vi "SensorTest-05-2017.vi"() -> ()   [LabVIEW 2010]
uses:
  <vilib>/userDefined/High Color/nirio_resource_hc.ctl
  <vilib>/rvi/interface/nirviOpenFPGA/nirviOpenFPGA.xnode
  C:/Users/HAGAR-IV/Desktop/Zeugs/markus/version feb 2012/FPGA Bitfiles/pertrasgcfpga2_FPGATarget_FPGA-TrapTest-05_C2F74D86.lvbitx
  C:/Users/HAGAR-IV/Desktop/Zeugs/Johnny/pertrasgc fpga/FPGA-TrapTest-05-2017.vi
  <vilib>/rvi/ClientSDK/nirviWhatTheDeviceIsDoing.ctl
  <vilib>/rvi/interface/nirviReadWriteControl/nirviReadWriteControl.xnode
  <vilib>/rvi/interface/common/niFpgaNodeNameForErrorReporting.ctl
  <vilib>/rvi/errors/niLvFpgaWhatHappensToTopLevelVI.ctl
  <vilib>/rvi/interface/nirviMethod/nirviMethod.xnode
  <vilib>/rvi/interface/nirviCloseFPGA/nirviCloseFPGA.xnode
  <vilib>/FPGAPlugInAG/cRIO-9114/niLvFpga_Open_cRIO-9114.vi
  <vilib>/Utility/error.llb/Error Cluster From Error Code.vi
  <vilib>/rvi/errors/niLvFpgaAdjustHostInterfaceError.vi
  <vilib>/FPGAPlugInAG/cRIO-9114/niLvFpga_Close_cRIO-9114.vi
  NiFpgaLv.dll
panel:
  out "MainCol2b":dbl format="%.23g"
  out "MainCol2a":dbl format="%.23g"
  out "MainCol1b":dbl format="%.23g"
  out "MainCol1a":dbl format="%.23g"
  out "PreCol2":dbl format="%.23g"
  out "PreCol1":dbl format="%.23g"
  out "Thermoelement":dbl format="%.23g"
  out "PTStirling":dbl format="%.23g"
  out "MesswertTrap2":dbl format="%.23g"
  out "MesswertTrap1":dbl format="%.23g"
  out "MesswertTrap2":dbl[](graph)
  out "MesswertTrap1":dbl[](graph)
  in  "Löschen":bool
  in  "Messwerte":i32=10
  in  "5Van(us)":u16=5500
  in  "Periode(us)":u32=100000
  in  "Warten(us)":u16=5000
  in  "zwischenMesswerten(us)":u16=10
  in  "stop":bool
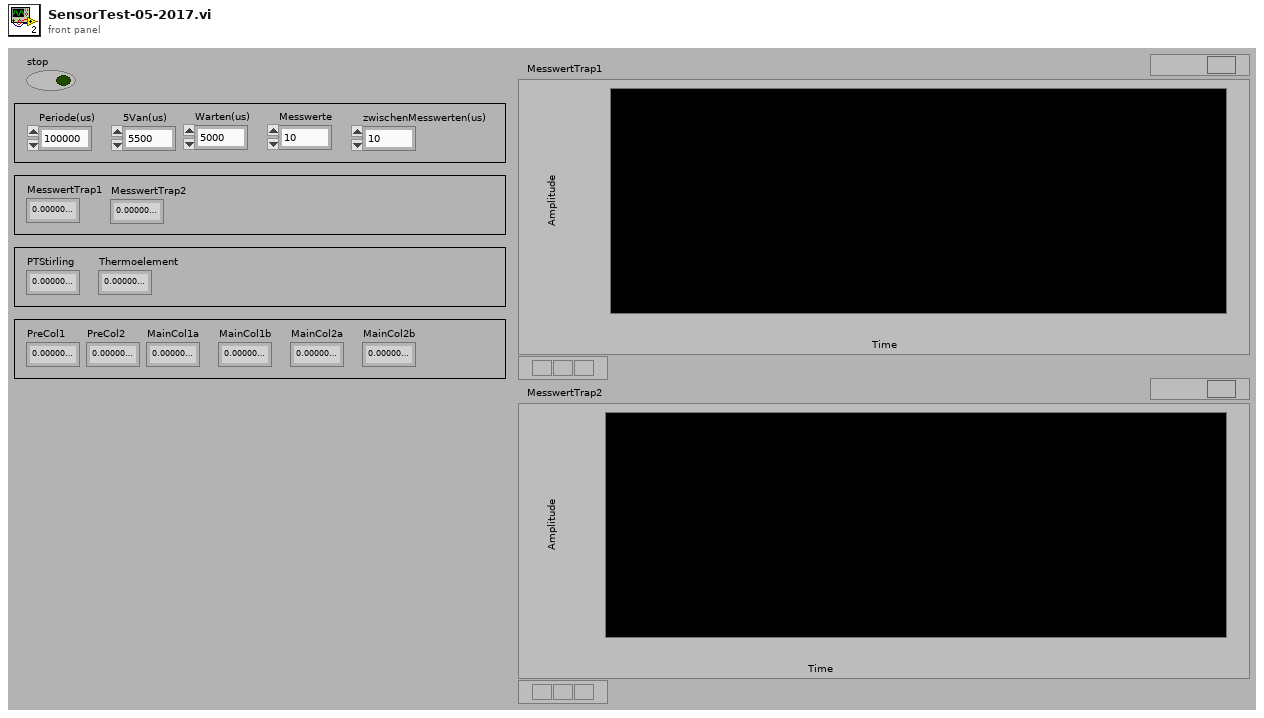
[diagram p1: front panel]
types:
  T1 = typedef "niFpgaNodeNameForErrorReporting.ctl" = enum16{"Open FPGA VI Reference", "Read/Write Control", "Invoke Method: Abort", "Invoke Method: Acknowledge IRQ", "Invoke Method: Download", "Invoke Method: FIFO.Configure", "Invoke Method: FIFO.Read", "Invoke Method: FIFO.Start", "Invoke Method: FIFO.Stop", "Invoke Method: FIFO.Write", "Invoke Method: Reset", "Invoke Method: Run", "Invoke Method: Wait on IRQ", "Close FPGA VI Reference"}
  T2 = typedef "niLvFpgaWhatHappensToTopLevelVI.ctl" = enum16{"top level VI scripted behind XNode", "top level VI inlined behind XNode"}
  T3 = cluster{"proportional gain (Kc)":fxp<+/-,16,8>, "integral gain (Kc*Ts/Ti)":fxp<+/-,16,8>, "derivative gain (Kc*Td/Ts)":fxp<+/-,16,8>}
  T4 = cluster{"[0]":dbl, "[1]":dbl, "[2]":dbl, "[3]":dbl, "[4]":dbl, "[5]":dbl, "[6]":dbl, "[7]":dbl, "[8]":dbl, "[9]":dbl}
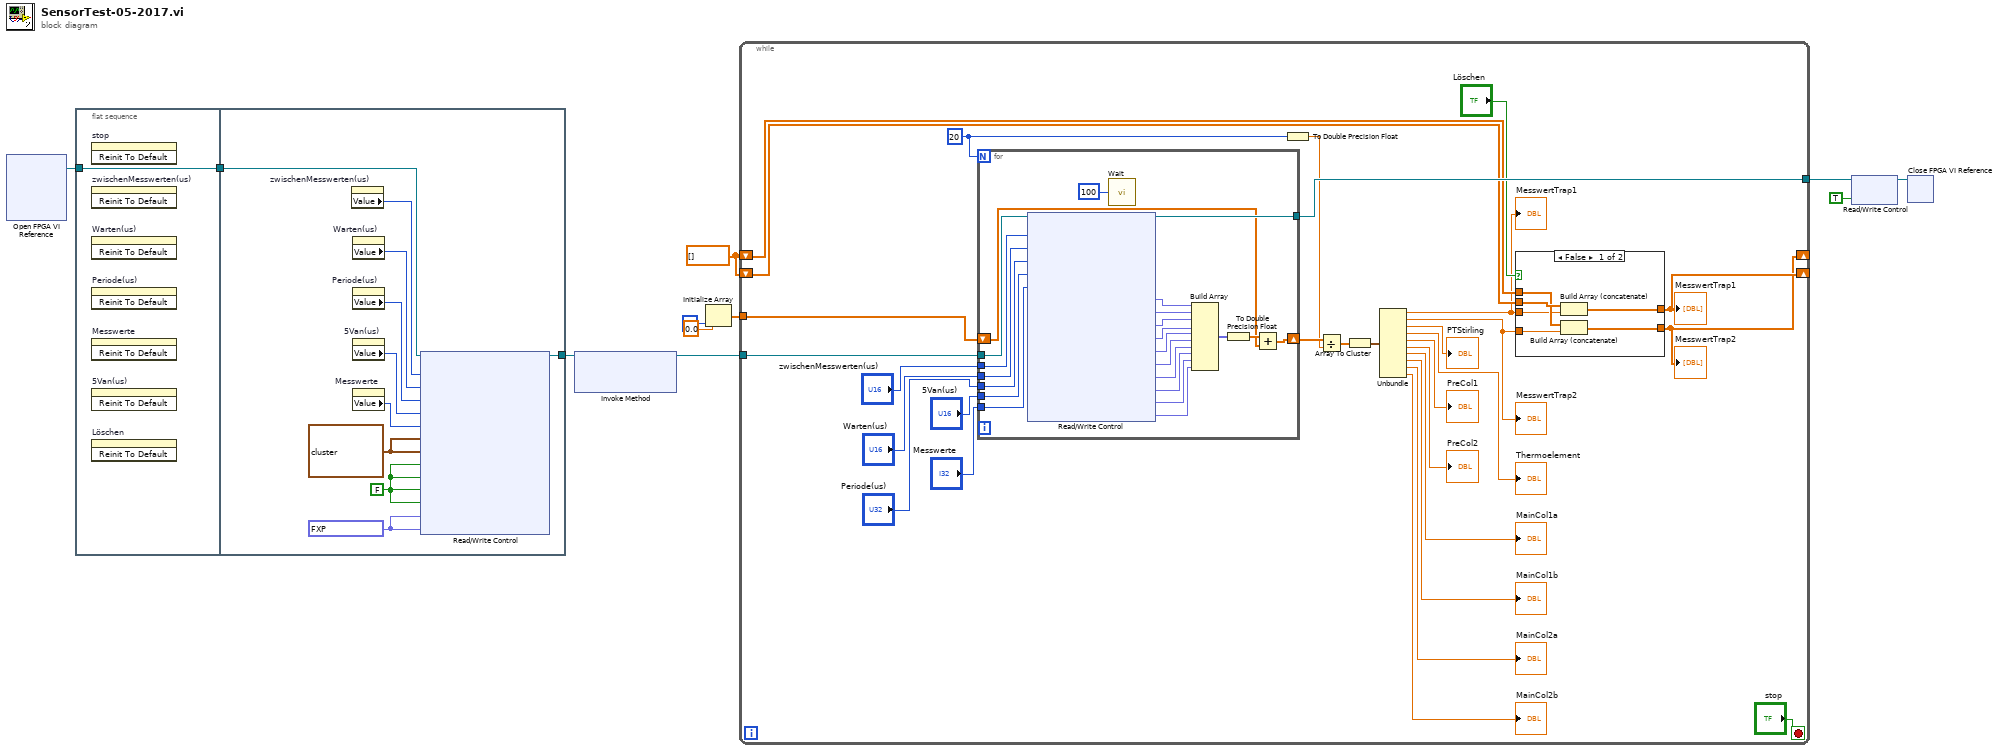
[diagram p0: block diagram]
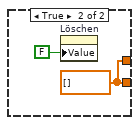
[diagram p2: hidden frame]
diagram:
  w4 = dbl[] []
  n1 = xnode "Open FPGA VI Reference"() -> ("FPGA VI Reference Out"=w11:refnum<k20>)  [unwired: 2 in, 1 out]
  n2 = flat-sequence {
    tunnel: w11 -> [w12]
    tunnel: [w12] -> w5
    tunnel: [w21] -> w10
    tunnel: w5 -> [w22]
    frame #0 {
      n3 = invoke on="stop" class="Bool (strict)" method="Reinit To Default"() -> ()  [unwired: 3 in, 3 out]
      n4 = invoke on="zwischenMesswerten(us)" class="DigNum (strict)" method="Reinit To Default"() -> ()  [unwired: 3 in, 3 out]
      n5 = invoke on="Warten(us)" class="DigNum (strict)" method="Reinit To Default"() -> ()  [unwired: 3 in, 3 out]
      n6 = invoke on="Periode(us)" class="DigNum (strict)" method="Reinit To Default"() -> ()  [unwired: 3 in, 3 out]
      n7 = invoke on="Messwerte" class="DigNum (strict)" method="Reinit To Default"() -> ()  [unwired: 3 in, 3 out]
      n8 = invoke on="5Van(us)" class="DigNum (strict)" method="Reinit To Default"() -> ()  [unwired: 3 in, 3 out]
      n9 = invoke on="Löschen" class="Bool (strict)" method="Reinit To Default"() -> ()  [unwired: 3 in, 3 out]
    }
    frame #1 {
      w13 = fxp<+/-,16,6> 0.0 ("setpointTrap1")
      w15 = T3 {"proportional gain (Kc)"=1.0, "integral gain (Kc*Ts/Ti)"=1.66796875, "derivative gain (Kc*Td/Ts)"=0.0} ("PIDTrap1")
      w14 = FALSE ("stop")
      n10 = property on="zwischenMesswerten(us)" class="DigNum (strict)"() -> ("Value"=w20:u16)  [unwired: 2 in, 2 out]
      n11 = property on="Warten(us)" class="DigNum (strict)"() -> ("Value"=w19:u16)  [unwired: 2 in, 2 out]
      n12 = property on="Periode(us)" class="DigNum (strict)"() -> ("Value"=w18:u32)  [unwired: 2 in, 2 out]
      n13 = property on="5Van(us)" class="DigNum (strict)"() -> ("Value"=w17:u16)  [unwired: 2 in, 2 out]
      n14 = property on="Messwerte" class="DigNum (strict)"() -> ("Value"=w16:i32)  [unwired: 2 in, 2 out]
      n15 = xnode "Read/Write Control"("FPGA VI Reference In"=w22, "zwischenMesswerten(us)"=w20, "Warten(us)"=w19, "Periode(us)"=w18, "5Van(us)"=w17, "Messwerte"=w16, "PIDTrap1"=w15, "PIDTrap2"=w15, "stop"=w14, "HeizenTrap1"=w14, "HeizenTrap2"=w14, "Stirling"=w14, "setpointTrap1"=w13, "setpointTrap2"=w13) -> ("FPGA VI Reference Out"=w21:refnum<k20>)  [unwired: 1 in, 1 out]
    }
  }
  n16 = xnode "Invoke Method"("FPGA VI Reference In"=w10) -> ("FPGA VI Reference Out"=w9:refnum<k20>)  [unwired: 2 in, 1 out]
  n17 = Initialize Array(0.0 ("element"), 10 ("dimension size")) -> (w1:dbl[])
  n18 = while {
    tunnel: w9 -> [w360]
    tunnel: [w358] -> w8
    shift-right: [w350] -> _
    shift-left: w4 -> [w352]
    shift-right: [w348] -> _
    shift-left: w4 -> [w349]
    tunnel: w1 -> [w332]
    stop <- "stop" stop-if-true
    w345 = 20
    n19 = for {
      N: w345 -> [_]
      tunnel: w360 -> [w382]
      tunnel: [w381] -> w358
      tunnel: "zwischenMesswerten(us)" -> [w380]
      tunnel: "Warten(us)" -> [w379]
      tunnel: "Periode(us)" -> [w378]
      tunnel: "5Van(us)" -> [w377]
      tunnel: "Messwerte" -> [w376]
      shift-right: [w363] -> w347
      shift-left: w332 -> [w361]
      n20 = xnode "Read/Write Control"("FPGA VI Reference In"=w382, "zwischenMesswerten(us)"=w380, "Warten(us)"=w379, "Periode(us)"=w378, "5Van(us)"=w377, "Messwerte"=w376) -> ("FPGA VI Reference Out"=w381:refnum<k20>, "MesswertTrap1"=w374:fxp<+/-,27,6>, "MesswertTrap2"=w373:fxp<+/-,27,6>, "PTStirling"=w372:fxp<+/-,26,5>, "Thermoelement"=w371:fxp<+/-,26,5>, "PreCol1"=w370:fxp<+/-,26,5>, "PreCol2"=w369:fxp<+/-,26,5>, "MainCol1a"=w368:fxp<+/-,26,5>, "MainCol1b"=w367:fxp<+/-,26,5>, "MainCol2a"=w366:fxp<+/-,26,5>, "MainCol2b"=w365:fxp<+/-,26,5>)  [unwired: 1 in, 1 out]
      n21 = call "Wait"("Count(mSec)"=u32 100) -> ()  [unwired: 1 out]
      n22 = Build Array(w374, w373, w372, w371, w370, w369, w368, w367, w366, w365) -> (w364:fxp<+/-,27,6>[])
      n23 = To Double Precision Float(number=w364) -> (double precision float=w362:dbl[])
      n24 = Add(x=w362, y=w361) -> (x+y=w363:dbl[])
    }
    n25 = To Double Precision Float(number=w345) -> (double precision float=w346:dbl)
    n26 = Divide(x=w347, y=w346) -> (x/y=w344:dbl[])
    n27 = Array To Cluster(array=w344) -> (cluster=w343:T4)
    n28 = Unbundle(w343) -> ("[0]"=w342:dbl, "[1]"=w341:dbl, "[2]"=→"PTStirling":dbl, "[3]"=→"Thermoelement":dbl, "[4]"=→"PreCol1":dbl, "[5]"=→"PreCol2":dbl, "[6]"=→"MainCol1a":dbl, "[7]"=→"MainCol1b":dbl, "[8]"=→"MainCol2a":dbl, "[9]"=→"MainCol2b":dbl)
    "MesswertTrap1" <- w342
    "MesswertTrap2" <- w341
    n29 = case shown="False" "Löschen" {
      tunnel: [w815 w816] -> w350
      tunnel: w352 -> [w814 _]
      tunnel: [w813 w816] -> w348
      tunnel: w349 -> [w812 _]
      tunnel: w342 -> [w811 _]
      tunnel: w341 -> [w810 _]
      frame False {
        n30 = Build Array (concatenate)(w814, w811) -> (w815:dbl[])
        n31 = Build Array (concatenate)(w812, w810) -> (w813:dbl[])
      }
      frame True {
        w816 = dbl[] []
        n32 = property on="Löschen" class="Bool (strict)"("Value"=FALSE ("Löschen")) -> ()  [unwired: 2 in, 2 out]
      }
    }
    "MesswertTrap1" <- w350
    "MesswertTrap2" <- w348
  }
  n33 = xnode "Read/Write Control"("FPGA VI Reference In"=w8, "stop"=TRUE) -> ("FPGA VI Reference Out"=w6:refnum<k20>)  [unwired: 1 in, 1 out]
  n34 = xnode "Close FPGA VI Reference"("FPGA VI Reference In"=w6) -> ()  [unwired: 1 in, 1 out]
